vi "RT Main.vi"() -> ()   [LabVIEW 2019]
uses:
  <vilib>/FPGAPlugInAG/ELVIS III/niLvFpga_Open_ELVIS III.vi
  <vilib>/rvi/interface/common/dynamic/niFpgaDynamicAddResources.vi
  <vilib>/Utility/error.llb/Error Cluster From Error Code.vi
  <vilib>/rvi/errors/niLvFpgaAdjustHostInterfaceError.vi
  <vilib>/rvi/interface/common/niFpgaWaitOnOcc.vi
  <vilib>/FPGAPlugInAG/Dynamic/niLvFpga_Run_Dynamic.vi
  <vilib>/FPGAPlugInAG/Dynamic/niLvFpga_Close_Dynamic.vi
  <vilib>/rvi/interface/nirviOpenFPGA/nirviOpenFPGA.xnode
  FPGA-Main.vi
  <vilib>/rvi/interface/nirviReadWriteControl/nirviReadWriteControl.xnode
  <vilib>/rvi/interface/nirviMethod/nirviMethod.xnode
  <vilib>/rvi/interface/nirviCloseFPGA/nirviCloseFPGA.xnode
  NiFpgaLv.dll
  <vilib>/rvi/interface/Simulation/niFpgaSimulationCallBeginRW.vi
  <vilib>/FPGAPlugInAG/Dynamic/niLvFpga_ConfigureFifo_Dynamic.vi
  <vilib>/rvi/errors/niLvFpgaMergeErrorWithErrorCode.vi
  <vilib>/FPGAPlugInAG/Dynamic/niLvFpga_ReadFifo_Dynamic.vi
panel:
  out "2k 频谱":waveform(dbl)(graph)
  out "1.5k 频谱":waveform(dbl)(graph)
  out "1k 4阶 频谱":waveform(dbl)(graph)
  out "1k 频谱":waveform(dbl)(graph)
  out "2k":waveform(dbl)(graph)
  out "1.5k":waveform(dbl)(graph)
  out "1k 4阶":waveform(dbl)(graph)
  out "1k":waveform(dbl)(graph)
  out "原始信号频谱":waveform(dbl)(graph)
  out "原始信号":waveform(dbl)(graph)
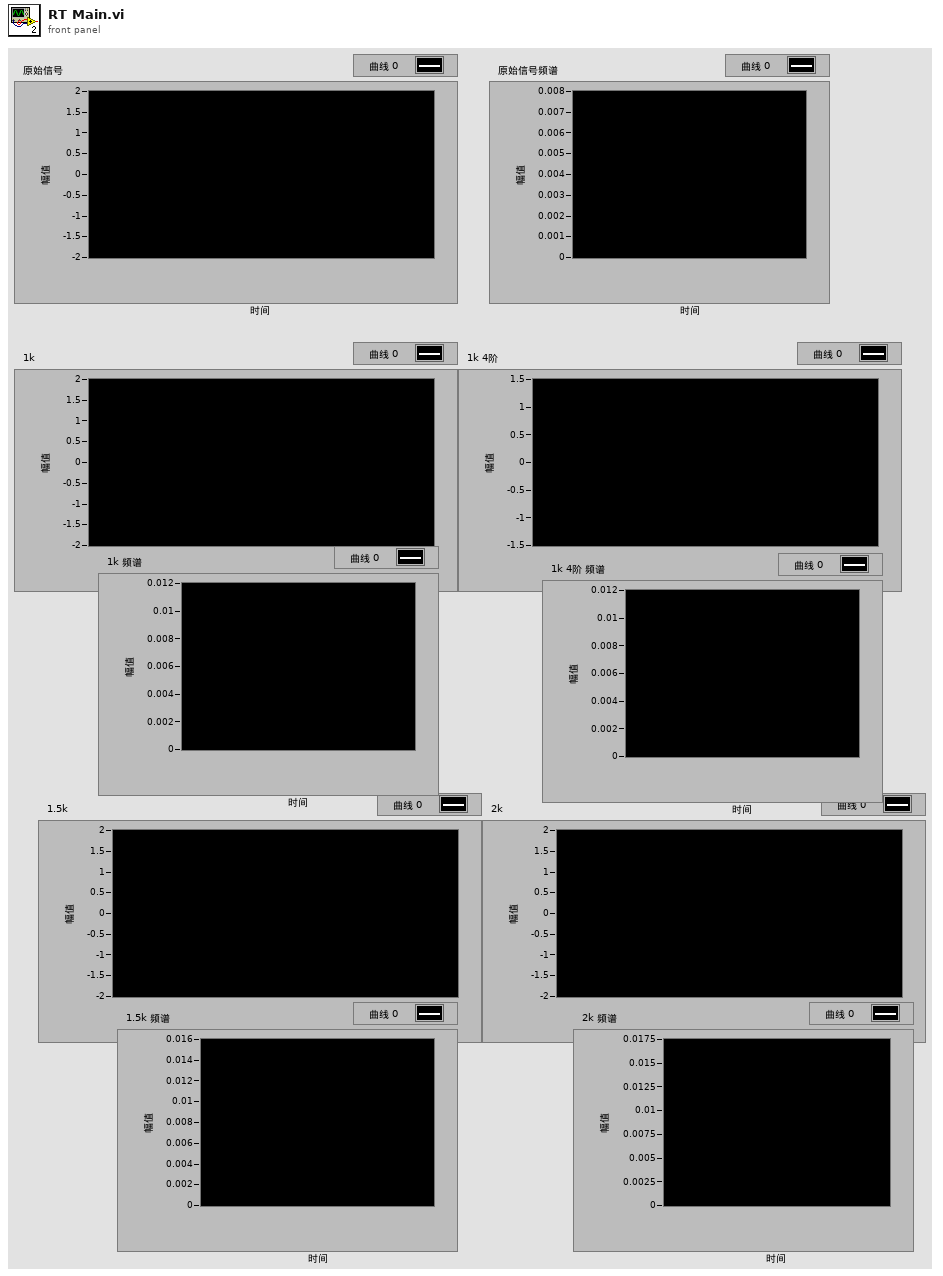
[diagram p1: front panel]
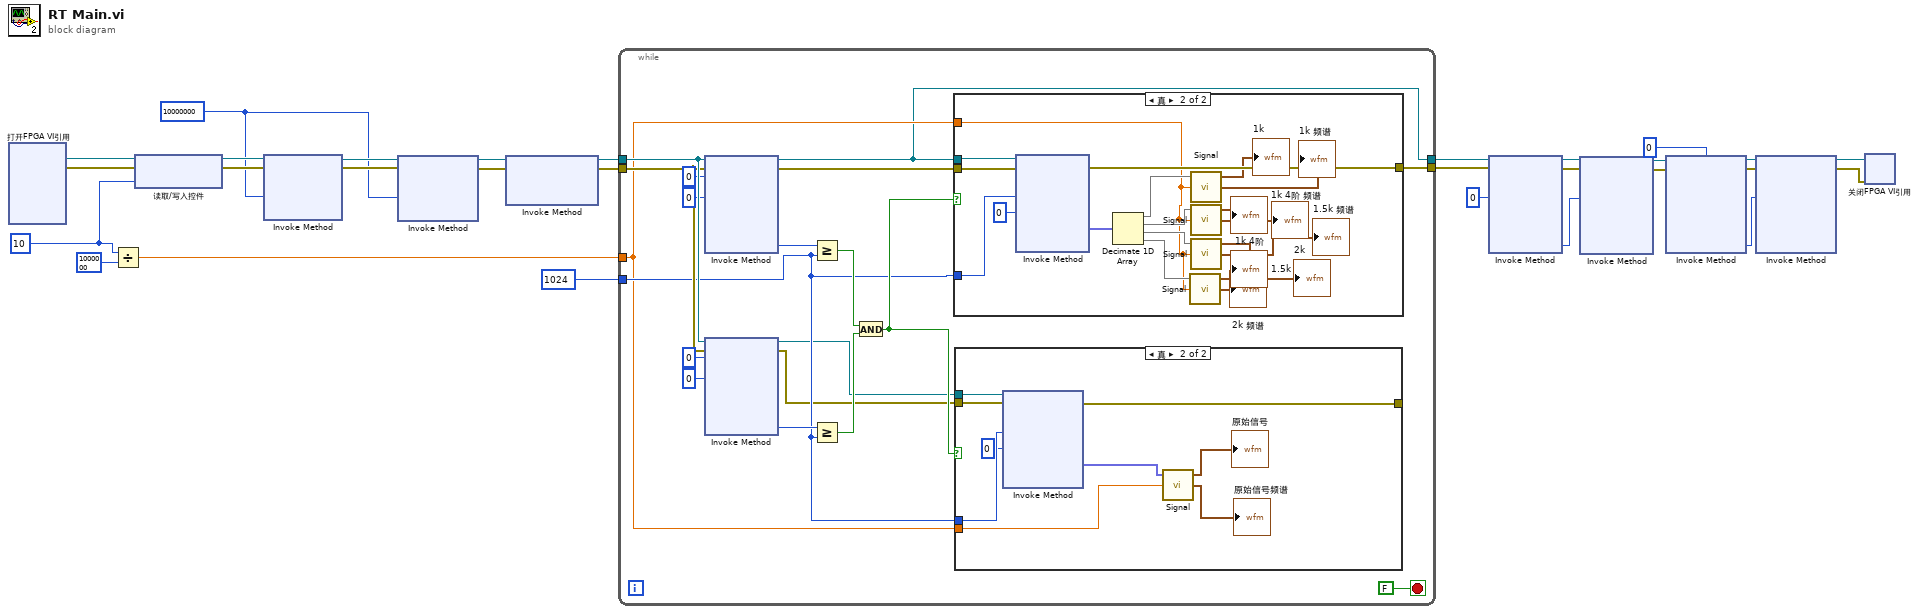
[diagram p0: block diagram]
diagram:
  w23 = u32 10000000 ("请求的深度")
  w17 = u32 10 ("Count(uSec)")
  n1 = xnode "打开FPGA VI引用"() -> ("FPGA VI引用输出"=w28:refnum<k20>, "错误输出"=w29:errorcluster)  [unwired: 2 in]
  n2 = Divide(x=w17, y=u32 1000000) -> (x/y=w15:dbl)
  n3 = xnode "读取/写入控件"("FPGA VI引用输入"=w28, "错误输入"=w29, "Count(uSec)"=w17) -> ("FPGA VI引用输出"=w26:refnum<k20>, "错误输出"=w27:errorcluster)
  n4 = xnode "Invoke Method"("FPGA VI引用输入"=w26, "错误输入"=w27, "请求的深度"=w23) -> ("FPGA VI引用输出"=w24:refnum<k20>, "错误输出"=w25:errorcluster)  [unwired: 1 out]
  n5 = xnode "Invoke Method"("FPGA VI引用输入"=w24, "错误输入"=w25, "请求的深度"=w23) -> ("FPGA VI引用输出"=w21:refnum<k20>, "错误输出"=w22:errorcluster)  [unwired: 1 out]
  n6 = xnode "Invoke Method"("FPGA VI引用输入"=w21, "错误输入"=w22) -> ("FPGA VI引用输出"=w19:refnum<k20>, "错误输出"=w20:errorcluster)  [unwired: 1 in]
  n7 = while {
    tunnel: w20 -> [w47]
    tunnel: w19 -> [w48]
    tunnel: u32 1024 -> [w37]
    tunnel: w15 -> [w33]
    tunnel: [w31] -> w14
    tunnel: [w30] -> w13
    stop <- FALSE stop-if-true
    n8 = xnode "Invoke Method"("FPGA VI引用输入"=w48, "错误输入"=w47, "元素数量"=u32 0, "超时(ms)"=0) -> ("FPGA VI引用输出"=w30:refnum<k20>, "错误输出"=w36:errorcluster, "剩余元素"=w40:u32)  [unwired: 1 out]
    n9 = xnode "Invoke Method"("FPGA VI引用输入"=w48, "错误输入"=w47, "元素数量"=u32 0, "超时(ms)"=0) -> ("FPGA VI引用输出"=w34:refnum<k20>, "错误输出"=w35:errorcluster, "剩余元素"=w39:u32)  [unwired: 1 out]
    n10 = Greater Or Equal?(x=w40, y=w37) -> (x >= y?=w42:bool)
    n11 = Greater Or Equal?(x=w39, y=w37) -> (x >= y?=w41:bool)
    n12 = And(x=w42, y=w41) -> (x .and. y?=w38:bool)
    n13 = case shown="真" w38 {
      tunnel: w37 -> [_ w76]
      tunnel: w36 -> [w59 w78]
      tunnel: w30 -> [_ w77]
      tunnel: [w59 w74] -> w31
      tunnel: w33 -> [_ w68]
      frame False {
      }
      frame True {
        n14 = xnode "Invoke Method"("FPGA VI引用输入"=w77, "错误输入"=w78, "元素数量"=w76, "超时(ms)"=0) -> ("错误输出"=w74:errorcluster, "数据"=w73:fxp<+/-,24,5>[])  [unwired: 2 out]
        n15 = Decimate 1D Array(w73) -> (w72:fxp<+/-,24,5>[], w71:fxp<+/-,24,5>[], w70:fxp<+/-,24,5>[], w69:fxp<+/-,24,5>[])
        n16 = call "Signal.vi"("dt"=w68, "数据"=w69) -> ("原始信号频谱"=→"2k 频谱":waveform(dbl), "原始信号"=→"2k":waveform(dbl))  [unwired: 1 in, 1 out]
        n17 = call "Signal.vi"("dt"=w68, "数据"=w72) -> ("原始信号频谱"=→"1k 频谱":waveform(dbl), "原始信号"=→"1k":waveform(dbl))  [unwired: 1 in, 1 out]
        n18 = call "Signal.vi"("dt"=w68, "数据"=w71) -> ("原始信号频谱"=→"1k 4阶 频谱":waveform(dbl), "原始信号"=→"1k 4阶":waveform(dbl))  [unwired: 1 in, 1 out]
        n19 = call "Signal.vi"("dt"=w68, "数据"=w70) -> ("原始信号频谱"=→"1.5k 频谱":waveform(dbl), "原始信号"=→"1.5k":waveform(dbl))  [unwired: 1 in, 1 out]
      }
    }
    n20 = case shown="真" w38 {
      tunnel: w37 -> [_ w55]
      tunnel: w35 -> [w49 w58]
      tunnel: w34 -> [_ w57]
      tunnel: [w49 w56] -> _
      tunnel: w33 -> [_ w52]
      frame False {
      }
      frame True {
        n21 = xnode "Invoke Method"("FPGA VI引用输入"=w57, "错误输入"=w58, "元素数量"=w55, "超时(ms)"=0) -> ("错误输出"=w56:errorcluster, "数据"=w53:fxp<+/-,24,5>[])  [unwired: 2 out]
        n22 = call "Signal.vi"("dt"=w52, "数据"=w53) -> ("原始信号频谱"=→"原始信号频谱":waveform(dbl), "原始信号"=→"原始信号":waveform(dbl))  [unwired: 1 in, 1 out]
      }
    }
  }
  n23 = xnode "Invoke Method"("FPGA VI引用输入"=w13, "错误输入"=w14, "元素数量"=u32 0) -> ("FPGA VI引用输出"=w12:refnum<k20>, "错误输出"=w11:errorcluster, "剩余元素"=w6:u32)  [unwired: 1 in, 1 out]
  n24 = xnode "Invoke Method"("FPGA VI引用输入"=w12, "错误输入"=w11, "元素数量"=w6) -> ("FPGA VI引用输出"=w10:refnum<k20>, "错误输出"=w9:errorcluster)  [unwired: 1 in, 2 out]
  n25 = xnode "Invoke Method"("FPGA VI引用输入"=w10, "错误输入"=w9, "元素数量"=u32 0) -> ("FPGA VI引用输出"=w8:refnum<k20>, "错误输出"=w7:errorcluster, "剩余元素"=w5:u32)  [unwired: 1 in, 1 out]
  n26 = xnode "Invoke Method"("FPGA VI引用输入"=w8, "错误输入"=w7, "元素数量"=w5) -> ("FPGA VI引用输出"=w2:refnum<k20>, "错误输出"=w1:errorcluster)  [unwired: 1 in, 2 out]
  n27 = xnode "关闭FPGA VI引用"("FPGA VI引用输入"=w2, "错误输入"=w1) -> ()  [unwired: 1 out]
